vi "Get Ball Pose.vi"(11 "Ball":refnum<class "Ball.lvclass">) -> (3 "Pose":T1)   [LabVIEW 2018]
uses:
  <vilib>/Analysis/Matrix/Datatypes/RealMatrix.ctl
  Ball_class/Ball.lvclass
  C:/Users/anton/Desktop/roboime/oop-vision/SSL_AI/Object_class/Object.lvclass
  Object_class/Object.lvclass/Object.ctl
  Object_class/Read x.vi
  Object_class/Read y.vi
  <vilib>/Analysis/Matrix/Numeric/Conversions/Array To Matrix - RA.vi
  <vilib>/Analysis/Matrix/NI_Matrix.lvlib
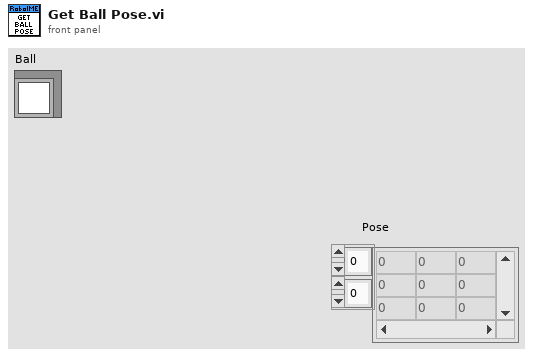
[diagram p1: front panel]
types:
  T1 = typedef "NI_Matrix.lvlib/RealMatrix.ctl" = dbl[][]
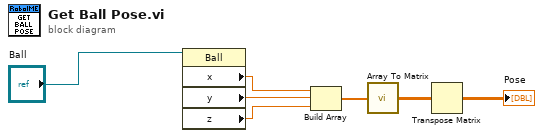
[diagram p0: block diagram]
diagram:
  n1 = property class="Ball"(reference="Ball") -> ("x"=w3:dbl, "y"=w2:dbl, "z"=w1:sgl)  [unwired: 1 in, 2 out]
  n2 = Build Array(w3, w2, w1) -> (w7:dbl[])
  n3 = call-poly <vilib>:"Array To Matrix.vi"("Real 1D Array"=w7) -> ("Real Matrix (Column Vector)"=w6:T1)
  n4 = Transpose Matrix(1:w6) -> (0:→"Pose":T1)
